vi "Read Zustandsgrössen.Hausmodell.vi"(8 "error in (no error)":errorcluster, 11 "Hausmodell in":refnum<class "Hausmodell.lvclass">) -> (0 "error out":errorcluster, 2 "Zustandsgrössen.Hausmodell":T1={"Raumtemperatur [°C]"=15.0, "Bodentemperatur [°C]"=15.0, "Rücklauftemperatur Heizkreislauf [°C]"=15.0}, 3 "Hausmodell out":refnum<class "Hausmodell.lvclass">)   [LabVIEW 2016, in "Hausmodell.lvclass"]
uses:
  Hausmodell.lvclass
  Hausmodell.lvclass/Hausmodell.ctl
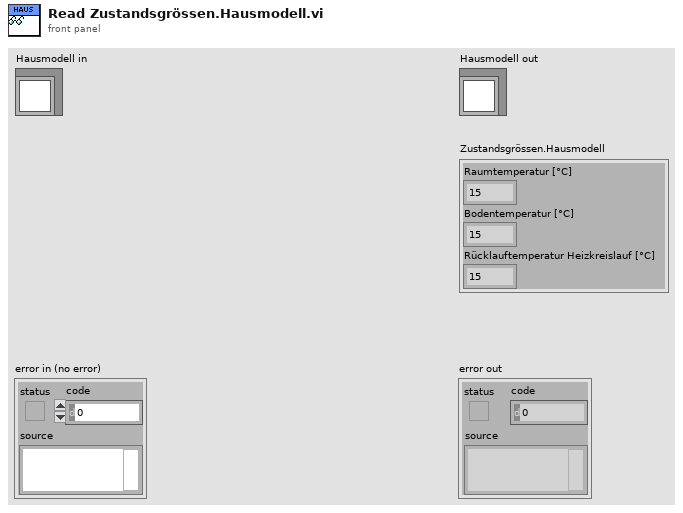
[diagram p1: front panel]
types:
  T1 = typedef "Hausmodell.lvclass/Hausmodell.Zustandsgrössen.ctl" = cluster{"Raumtemperatur [°C]":dbl, "Bodentemperatur [°C]":dbl, "Rücklauftemperatur Heizkreislauf [°C]":dbl}
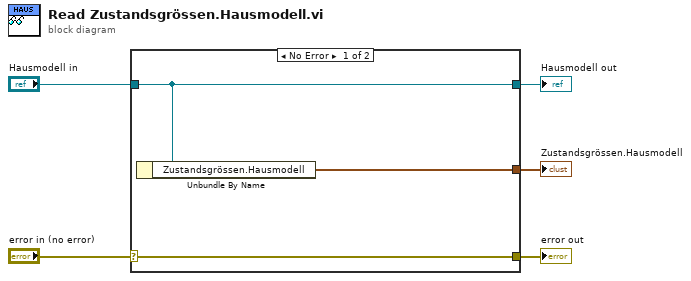
[diagram p0: block diagram]
diagram:
  n1 = case shown="No Error" "error in (no error)" {
    selector: "error in (no error)" -> [w8 w9]
    tunnel: [w8 w9] -> w4
    tunnel: [w7 w10] -> w2
    tunnel: "Hausmodell in" -> [w7 w10]
    tunnel: [w6 _] -> w1
    frame No Error {
      n2 = Unbundle By Name(w7) -> ("Zustandsgrössen.Hausmodell"=w6:T1)
    }
    frame Error {
    }
  }
  "error out" <- w4
  "Hausmodell out" <- w2
  "Zustandsgrössen.Hausmodell" <- w1
